vi "Add Terminals.vi"(6 "acyclic frame names":string[](array[string]), 8 "error in":errorcluster, 10 "terminals":T2[](array[typedef]), 11 "port in":T1 format="%.0x") -> (0 "error out":errorcluster, 3 "port out":T1 format="%.0x")   [LabVIEW 2020, in "Ballard MIL-STD-1553 Scripting.lvlib"]
uses:
  Ballard MIL-STD-1553 Scripting.lvlib
  Shared/Terminal Name and Address.ctl
  Shared/Address.ctl
  <vilib>/NI VeriStand/Custom Device API/Custom Device Item Ref.ctl
  <vilib>/NI VeriStand/Custom Device API/Custom Device API.lvlib
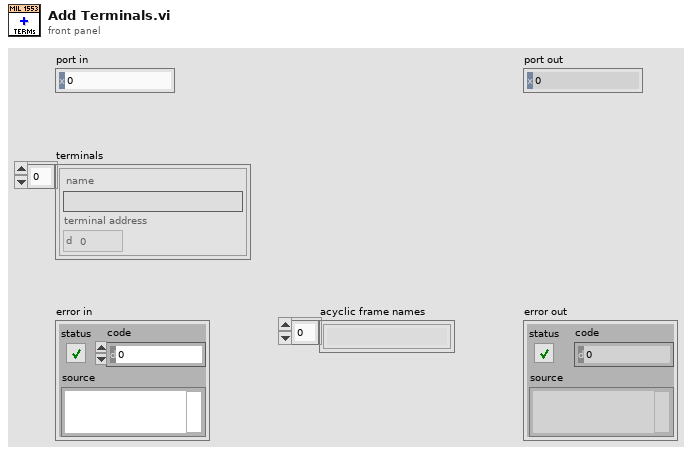
[diagram p1: front panel]
types:
  T1 = typedef "Custom Device API.lvlib/Custom Device Item Ref.ctl" = u64
  T2 = typedef "Terminal Name and Address.ctl" = cluster{"name":string, "terminal address":T3}
  T3 = typedef "Address.ctl" = u16
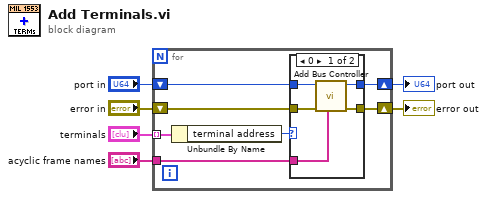
[diagram p0: block diagram]
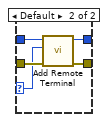
[diagram p2: hidden frame]
diagram:
  n1 = for {
    shift-right: [w9] -> w2
    shift-left: "error in" -> [w10]
    tunnel: "terminals" -> [w13] mode=indexing
    tunnel: "acyclic frame names" -> [w8]
    shift-right: [w7] -> w3
    shift-left: "port in" -> [w11]
    n2 = Unbundle By Name(w13) -> ("terminal address"=w12:T3)
    n3 = case shown="0" w12 {
      selector: w12 -> [_ w20]
      tunnel: w11 -> [w18 w21]
      tunnel: w10 -> [w17 w23]
      tunnel: [w16 w22] -> w9
      tunnel: w8 -> [w14 _]
      tunnel: [w15 w19] -> w7
      frame 0 {
        n4 = call "Add Bus Controller.vi"("acyclic frame names"=w14, "error in"=w17, "port in"=w18) -> ("error out"=w16:errorcluster, "port out"=w15:T1)  [unwired: 6 in, 1 out]
      }
      frame Default {
        n5 = call "Add Remote Terminal.vi"("error in"=w23, "terminal address"=w20, "port in"=w21) -> ("error out"=w22:errorcluster, "port out"=w19:T1)  [unwired: 6 in, 1 out]
      }
    }
  }
  "port out" <- w3
  "error out" <- w2
